vi "Deep Copy.vi"(8 "error in (no error)":errorcluster, 11 "Result Model in":refnum<class "Result Model.lvclass">) -> (0 "error out":errorcluster, 2 "Result Model Copy":refnum<class "Result Model.lvclass">)   [LabVIEW 2020, in "Result Model.lvclass"]
uses:
  Result Model.lvclass
  Result Model.lvclass/Result Model.ctl
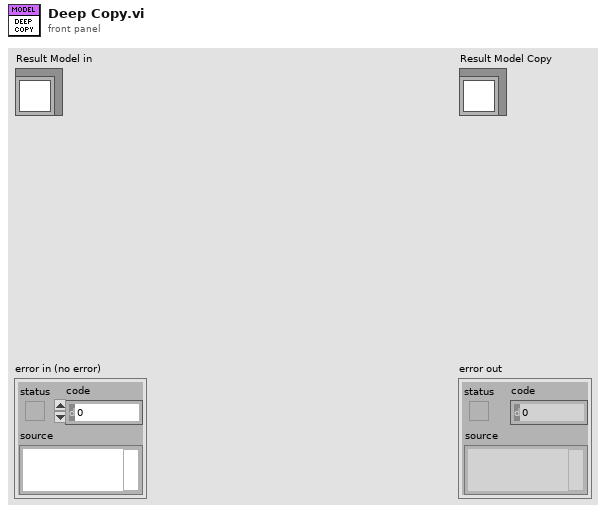
[diagram p1: front panel]
types:
  T1 = typedef "Result Model.lvclass/Model State.ctl" = cluster{"Run Queue":set{string}, "Test Statuses":map{string, T2}, "Execution Time":map{string, dbl}, "Assertions":map{string, cluster{"Result Type":T3, "Status":T2, "Message":string, "Description":string}[]}}
  T2 = typedef "Result.lvlib/Status.ctl" = enum16{"", "Passed", "Failed", "Error", "Skipped", "Setup Error", "Broken", "Teardown Error"}
  T3 = typedef "Result.lvlib/Type.ctl" = enum16{"Method", "Case", "Suite", "Pass", "Fail", "Skip", "Pass if", "Fail if", "Pass if Error", "Fail if Error", "Pass if Equal", "Fail if Equal"}
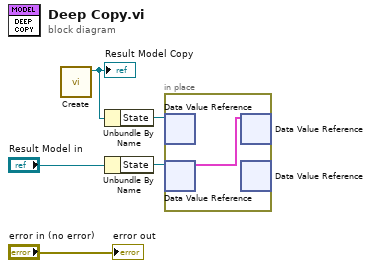
[diagram p0: block diagram]
diagram:
  n1 = call "Create.vi"() -> ("Result Model out"=w3:refnum<class "Result Model.lvclass">)  [unwired: 11 in]
  "Result Model Copy" <- w3
  n2 = Unbundle By Name(w3) -> ("State"=w1:refnum<data-value>)
  n3 = Unbundle By Name("Result Model in") -> ("State"=w2:refnum<data-value>)
  n4 = in-place {
    n5 = in-place-dvr #1(w1) -> ()  [unwired: 2 out]
    n6 = in-place-dvr #2(w2) -> (w6:T1)  [unwired: 1 out]
    n7 = in-place-dvr #1(w6) -> ()  [unwired: 2 out]
    n8 = in-place-dvr #2() -> ()  [unwired: 1 in, 2 out]
  }
  "error out" <- "error in (no error)"
